vi "PID_controller_00.vi"() -> ()   [LabVIEW 2011]
panel:
  out "Process value":dbl
  in  "stop":bool
  out "prev error":dbl
  out "derivative":dbl
  in  "integral":dbl
  out "error":dbl
  out "Current angle (deg)":dbl
  in  "Kd":dbl
  in  "Ki":dbl
  in  "Kp":dbl
  out "Current value (torr)":dbl
  in  "Set Point (torr)":dbl
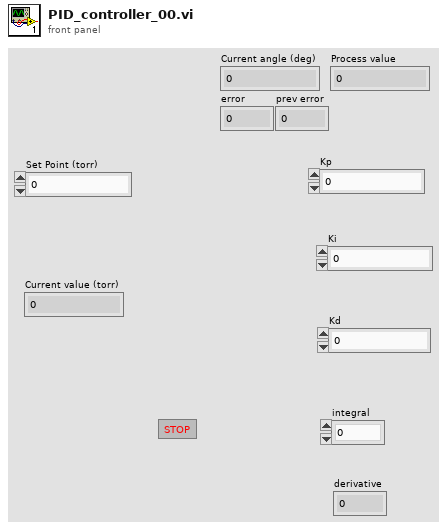
[diagram p1: front panel]
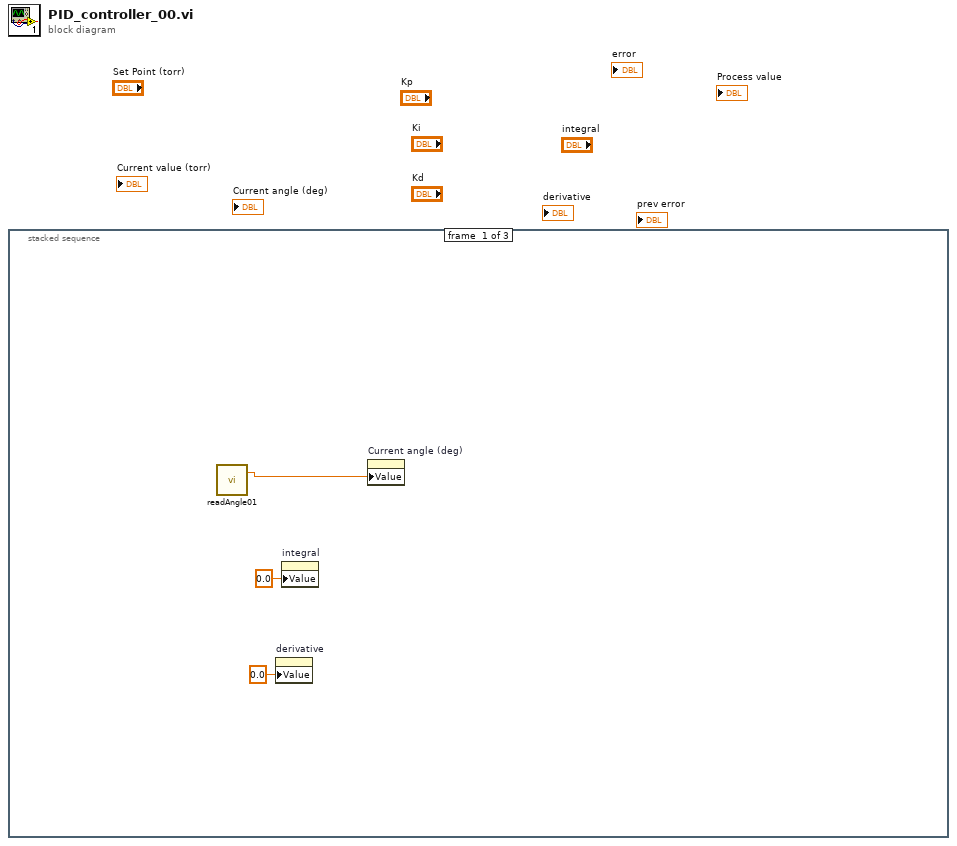
[diagram p0: block diagram]
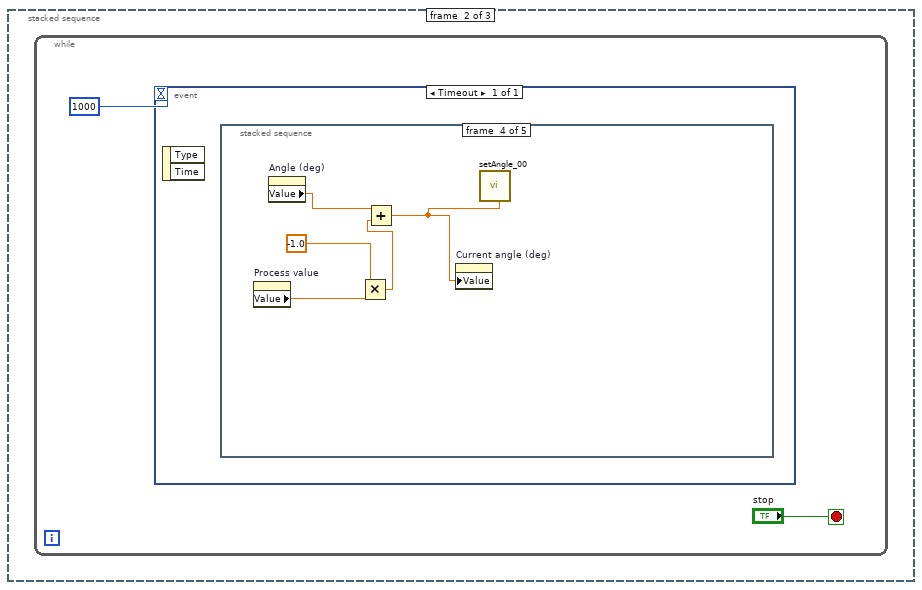
[diagram p2: hidden frame]
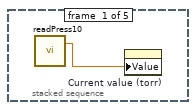
[diagram p3: hidden frame]
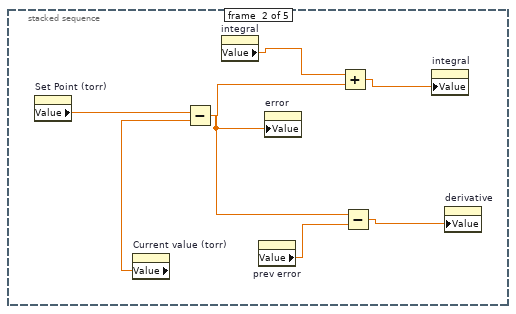
[diagram p4: hidden frame]
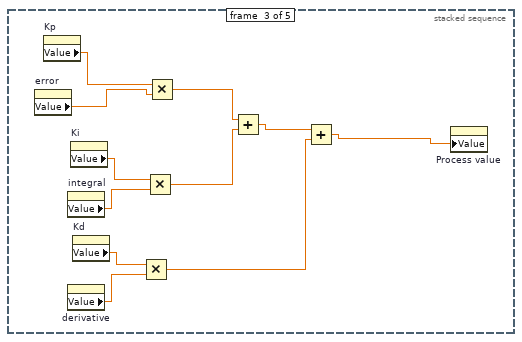
[diagram p5: hidden frame]
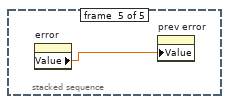
[diagram p6: hidden frame]
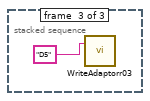
[diagram p7: hidden frame]
diagram:
  n1 = stacked-sequence {
    frame #0 {
      n2 = call "readAngle01.vi"() -> ("angle"=w3:dbl)  [unwired: 1 in, 1 out]
      n3 = property on="derivative" class="DigNum (strict)"("Value"=0.0 ("derivative")) -> ()  [unwired: 2 in, 2 out]
      n4 = property on="integral" class="DigNum (strict)"("Value"=0.0 ("integral")) -> ()  [unwired: 2 in, 2 out]
      n5 = property on="Current angle (deg)" class="DigNum (strict)"("Value"=w3) -> ()  [unwired: 2 in, 2 out]
    }
    frame #1 {
      n6 = while {
        stop <- "stop" stop-if-true
        n7 = event shown="[0] Timeout" {
          selector: _ -> [_]
          dyn-events: _ -> [_]
          timeout: 1000 -> [_]
          event Timeout {
            n8 = event-data() -> ()  [unwired: 1 in, 2 out]
            n9 = stacked-sequence {
              frame #0 {
                n10 = call "readPress10.vi"() -> ("P"=w6:dbl)  [unwired: 1 in, 1 out]
                n11 = property on="Current value (torr)" class="DigNum (strict)"("Value"=w6) -> ()  [unwired: 2 in, 2 out]
              }
              frame #1 {
                n12 = property on="Set Point (torr)" class="DigNum (strict)"() -> ("Value"=w7:dbl)  [unwired: 2 in, 2 out]
                n13 = property on="Current value (torr)" class="DigNum (strict)"() -> ("Value"=w8:dbl)  [unwired: 2 in, 2 out]
                n14 = Subtract(x=w7, y=w8) -> (x-y=w9:dbl)
                n15 = property on="integral" class="DigNum (strict)"() -> ("Value"=w13:dbl)  [unwired: 2 in, 2 out]
                n16 = property on="prev error" class="DigNum (strict)"() -> ("Value"=w10:dbl)  [unwired: 2 in, 2 out]
                n17 = property on="error" class="DigNum (strict)"("Value"=w9) -> ()  [unwired: 2 in, 2 out]
                n18 = Add(x=w13, y=w9) -> (x+y=w12:dbl)
                n19 = Subtract(x=w9, y=w10) -> (x-y=w11:dbl)
                n20 = property on="integral" class="DigNum (strict)"("Value"=w12) -> ()  [unwired: 2 in, 2 out]
                n21 = property on="derivative" class="DigNum (strict)"("Value"=w11) -> ()  [unwired: 2 in, 2 out]
              }
              frame #2 {
                n22 = property on="error" class="DigNum (strict)"() -> ("Value"=w24:dbl)  [unwired: 2 in, 2 out]
                n23 = property on="Kp" class="DigNum (strict)"() -> ("Value"=w23:dbl)  [unwired: 2 in, 2 out]
                n24 = property on="integral" class="DigNum (strict)"() -> ("Value"=w21:dbl)  [unwired: 2 in, 2 out]
                n25 = property on="derivative" class="DigNum (strict)"() -> ("Value"=w19:dbl)  [unwired: 2 in, 2 out]
                n26 = property on="Ki" class="DigNum (strict)"() -> ("Value"=w22:dbl)  [unwired: 2 in, 2 out]
                n27 = property on="Kd" class="DigNum (strict)"() -> ("Value"=w20:dbl)  [unwired: 2 in, 2 out]
                n28 = Multiply(x=w20, y=w19) -> (x*y=w16:dbl)
                n29 = Multiply(x=w22, y=w21) -> (x*y=w17:dbl)
                n30 = Multiply(x=w23, y=w24) -> (x*y=w18:dbl)
                n31 = Add(x=w18, y=w17) -> (x+y=w15:dbl)
                n32 = Add(x=w15, y=w16) -> (x+y=w14:dbl)
                n33 = property on="Process value" class="DigNum (strict)"("Value"=w14) -> ()  [unwired: 2 in, 2 out]
              }
              frame #3 {
                n34 = property on="Process value" class="DigNum (strict)"() -> ("Value"=w27:dbl)  [unwired: 2 in, 2 out]
                n35 = property on="Angle (deg)" class="DigNum (strict)"() -> ("Value"=w29:dbl)  [unwired: 2 in, 2 out]
                n36 = Multiply(x=-1.0, y=w27) -> (x*y=w25:dbl)
                n37 = Add(x=w29, y=w25) -> (x+y=w28:dbl)
                n38 = property on="Current angle (deg)" class="DigNum (strict)"("Value"=w28) -> ()  [unwired: 2 in, 2 out]
                n39 = call "setAngle_00.vi"("Angle (deg)"=w28) -> ()  [unwired: 1 in, 1 out]
              }
              frame #4 {
                n40 = property on="error" class="DigNum (strict)"() -> ("Value"=w30:dbl)  [unwired: 2 in, 2 out]
                n41 = property on="prev error" class="DigNum (strict)"("Value"=w30) -> ()  [unwired: 2 in, 2 out]
              }
            }
          }
        }
      }
    }
    frame #2 {
      n42 = call "WriteAdaptorr03.vi"("string to write"="D5") -> ()  [unwired: 1 in, 1 out]
    }
  }
